vi "OAT Track Orders in Resampled Signal.vi"   [LabVIEW 2017]
doc: "Computes magnitudes and phases for designated orders from <B>resampled signal</B>."
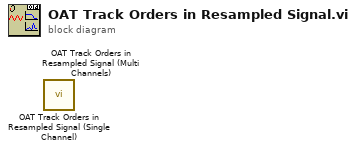
[diagram p0: block diagram]
diagram:
  n1 = call <vilib>:"OAT Track Orders in Resampled Signal (Single Channel).vi"() -> ()  [unwired: 11 in, 5 out]
  n2 = call <vilib>:"OAT Track Orders in Resampled Signal (Multi Channels).vi"() -> ()  [unwired: 11 in, 5 out]
